vi "LaserLineDetection_Intensity_ImageCenter.vi"(11 "Camera Parameters":T1) -> (3 "Image Center (Horizontal)":i32)   [LabVIEW 2013]
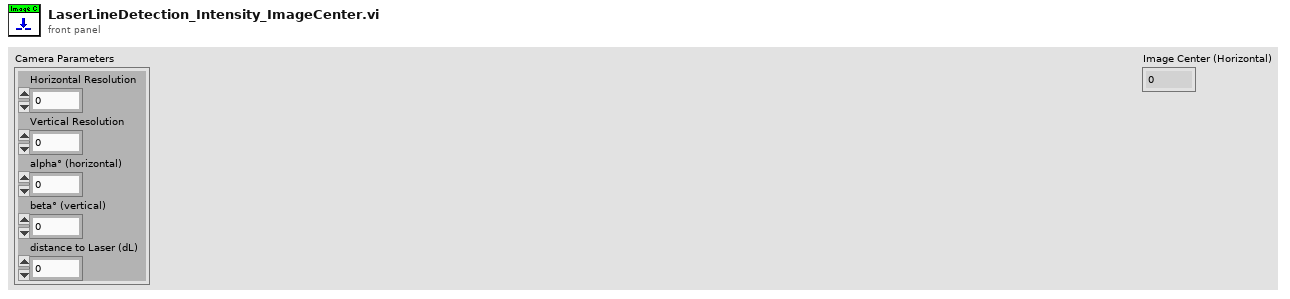
[diagram p1: front panel]
types:
  T1 = cluster{"Horizontal Resolution":dbl, "Vertical Resolution":dbl, "alpha° (horizontal)":dbl, "beta° (vertical)":dbl, "distance to Laser (dL)":dbl}
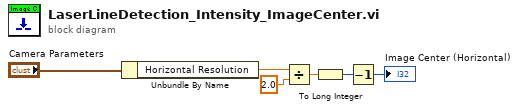
[diagram p0: block diagram]
diagram:
  n1 = Unbundle By Name("Camera Parameters") -> ("Horizontal Resolution"=w5:dbl)
  n2 = Divide(x=w5, y=2.0) -> (x/y=w2:dbl)
  n3 = To Long Integer(number=w2) -> (32bit integer=w3:i32)
  n4 = Decrement(x=w3) -> (x-1=→"Image Center (Horizontal)":i32)
